vi "get settings string.vi"(11 "VI in":refnum<vi>) -> (0 "error out":errorcluster, 3 "Settings string":string)   [LabVIEW 2016, in "SaveLoad.lvlib"]
doc: "Creates text string of control names and values to be saved. Output can be put into a pop up or saved directly to file"
uses:
  SaveLoad.lvlib
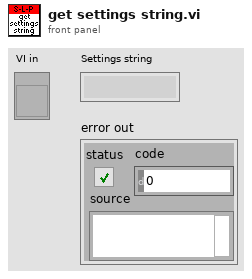
[diagram p1: front panel]
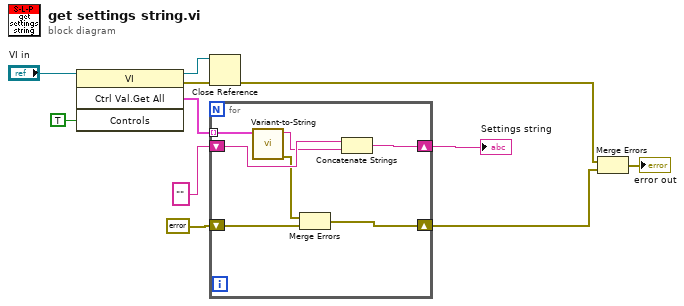
[diagram p0: block diagram]
diagram:
  n1 = invoke class="VI" method="Ctrl Val.Get All"(reference="VI in", "Controls"=TRUE) -> (reference out=w3:refnum<vi>, error out=w4:errorcluster, "Get All Control Values Variant"=w6:cluster{"Name":string, "Variant Data":variant}[])  [unwired: 2 in, 1 out]
  n2 = Close Reference(reference=w3, error in (no error)=w4) -> (error out=w5:errorcluster)
  n3 = for {
    tunnel: w6 -> [w14] mode=indexing
    shift-right: [w18] -> w8
    shift-left: "" -> [w17]
    shift-right: [w16] -> w11
    shift-left: errorcluster {"status"=FALSE, "code"=0, "source"=""} ("error IO") -> [w15]
    n4 = call "Variant-to-String.vi"("Cluster"=w14) -> ("error out"=w12:errorcluster, "String"=w13:string)  [unwired: 9 in]
    n5 = Merge Errors(w12, w15) -> (w16:errorcluster)
    n6 = Concatenate Strings(w17, w13) -> (w18:string)
  }
  "Settings string" <- w8
  n7 = Merge Errors(w5, w11) -> (→"error out":errorcluster)
